vi "power_monitor.vi"(0 "IP / Hostname":string="172.20.125.112") -> (4 "voltage":dbl, 6 "frequency":dbl, 8 "apparant power (watt)":i32, 10 "active power (watt)":i32, 15 "power factor":dbl)   [LabVIEW 2021]
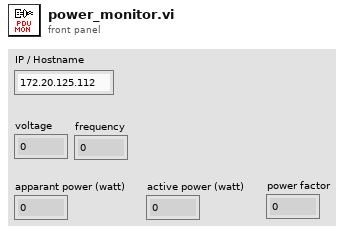
[diagram p1: front panel]
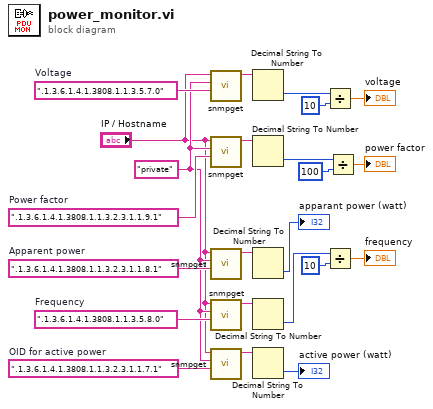
[diagram p0: block diagram]
diagram:
  w19 = ".1.3.6.1.4.1.3808.1.1.3.5.8.0"  # Frequency
  w20 = ".1.3.6.1.4.1.3808.1.1.3.5.7.0"  # Voltage
  w21 = ".1.3.6.1.4.1.3808.1.1.3.2.3.1.1.9.1"  # Power factor
  w22 = ".1.3.6.1.4.1.3808.1.1.3.2.3.1.1.8.1"  # Apparent power
  w23 = ".1.3.6.1.4.1.3808.1.1.3.2.3.1.1.7.1"  # OID for active power
  w18 = "private" ("community")
  n1 = call "snmpget.vi"("OID"=w20, "community"=w18, "IP / Hostname"="IP / Hostname") -> ("return"=w1:string)  [unwired: 7 in, 1 out]
  n2 = call "snmpget.vi"("OID"=w21, "community"=w18, "IP / Hostname"="IP / Hostname") -> ("return"=w12:string)  [unwired: 7 in, 1 out]
  n3 = call "snmpget.vi"("OID"=w22, "community"=w18, "IP / Hostname"="IP / Hostname") -> ("return"=w13:string)  [unwired: 7 in, 1 out]
  n4 = call "snmpget.vi"("OID"=w19, "community"=w18, "IP / Hostname"="IP / Hostname") -> ("return"=w5:string)  [unwired: 7 in, 1 out]
  n5 = call "snmpget.vi"("OID"=w23, "community"=w18, "IP / Hostname"="IP / Hostname") -> ("return"=w16:string)  [unwired: 7 in, 1 out]
  n6 = Decimal String To Number(string=w1) -> (number=w4:i32)  [unwired: 2 in, 1 out]
  n7 = Decimal String To Number(string=w12) -> (number=w11:i32)  [unwired: 2 in, 1 out]
  n8 = Decimal String To Number(string=w13) -> (number=→"apparant power (watt)":i32)  [unwired: 2 in, 1 out]
  n9 = Decimal String To Number(string=w5) -> (number=w6:i32)  [unwired: 2 in, 1 out]
  n10 = Decimal String To Number(string=w16) -> (number=→"active power (watt)":i32)  [unwired: 2 in, 1 out]
  n11 = Divide(x=w4, y=10) -> (x/y=→"voltage":dbl)
  n12 = Divide(x=w6, y=10) -> (x/y=→"frequency":dbl)
  n13 = Divide(x=w11, y=100) -> (x/y=→"power factor":dbl)
